vi "Gear_Components.vi"(9 "Target Seperation":dbl, 10 "Far Target Distance":dbl, 11 "Close Target Distance":dbl) -> (2 "Y Component":dbl, 3 "X Component":dbl)   [LabVIEW 2016]
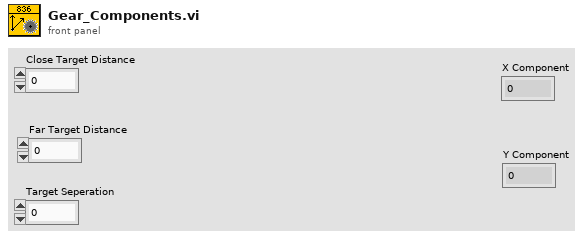
[diagram p1: front panel]
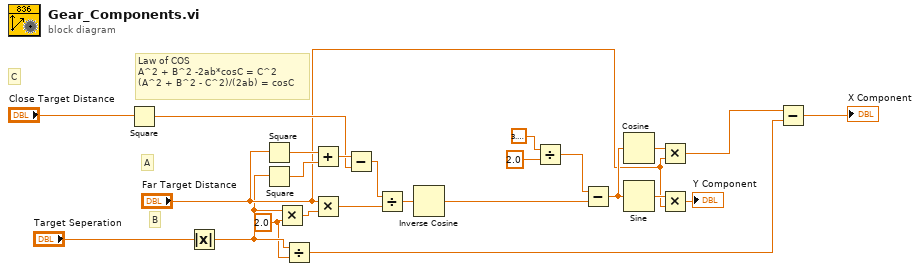
[diagram p0: block diagram]
diagram:
  w4 = 2.0 ("y")
  # "B"
  # "A"
  # "C"
  # "Law of COS\nA^2 + B^2 -2ab*cosC = C^2\n(A^2 + B^2 - C^2)/(2ab) = cosC"
  n1 = Square(x="Close Target Distance") -> (x^2=w20:dbl)
  n2 = Absolute Value(x="Target Seperation") -> (abs(x)=w5:dbl)
  n3 = Square(x="Far Target Distance") -> (x^2=w23:dbl)
  n4 = Square(x=w5) -> (x^2=w22:dbl)
  n5 = Multiply(x=w5, y=w4) -> (x*y=w19:dbl)
  n6 = Divide(x=w5, y=w4) -> (x/y=w2:dbl)
  n7 = Add(x=w23, y=w22) -> (x+y=w21:dbl)
  n8 = Multiply(x="Far Target Distance", y=w19) -> (x*y=w18:dbl)
  n9 = Subtract(x=w21, y=w20) -> (x-y=w17:dbl)
  n10 = Divide(x=w17, y=w18) -> (x/y=w16:dbl)
  n11 = Inverse Cosine(1:w16) -> (0:w15:dbl)
  n12 = Divide(x=3.141592653589793, y=2.0) -> (x/y=w7:dbl)
  n13 = Subtract(x=w7, y=w15) -> (x-y=w14:dbl)
  n14 = Cosine(x=w14) -> (cos(x)=w12:dbl)
  n15 = Sine(x=w14) -> (sin(x)=w13:dbl)
  n16 = Multiply(x=w12, y="Far Target Distance") -> (x*y=w3:dbl)
  n17 = Multiply(x=w13, y="Far Target Distance") -> (x*y=→"Y Component":dbl)
  n18 = Subtract(x=w3, y=w2) -> (x-y=→"X Component":dbl)
